vi "SetGlobalToZero.vi"(11 "subwindow control":T2={"2^n : x"=10, "2^n : y"=10, "lower left box Position"={"X"=1752.0, "Y"=1167.0}, "Height"=0, "Width"=0} {"Width" min=32 max=4704; "Height" min=2 max=3424; "2^n : y" min=1 max=13; "2^n : x" min=1 max=13}) -> ()   [LabVIEW 2018]
uses:
  <vilib>/Utility/miscctls.llb/LVPointDoubleTypeDef.ctl
  References.vi
  General Libraries/Photon Filtering.lvlib
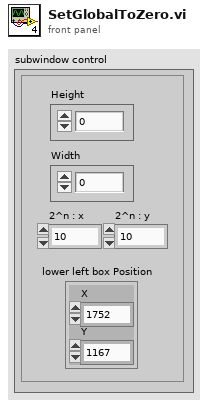
[diagram p1: front panel]
types:
  T1 = typedef "LVPointDoubleTypeDef.ctl" = cluster{"X":dbl, "Y":dbl}
  T2 = cluster{"2^n : x":i8, "2^n : y":i8, "lower left box Position":T1, "Height":i32, "Width":i32}
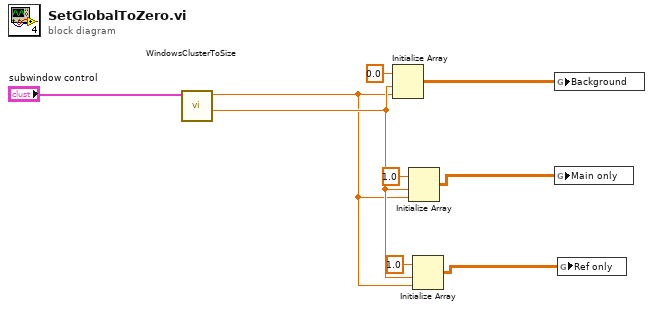
[diagram p0: block diagram]
diagram:
  n1 = call "WindowsClusterToSize.vi"("subwindow control 2"="subwindow control") -> ("Ny"=w6:dbl, "Nx"=w5:dbl)  [unwired: 9 in]
  n2 = Initialize Array(0.0 ("element"), w6, w5) -> (w7:dbl[][])
  n3 = Initialize Array "Initialize Array"(1.0 ("element"), w6, w5) -> (w2:dbl[][])
  n4 = Initialize Array "Initialize Array"(1.0 ("element"), w6, w5) -> (w1:dbl[][])
  n5 = global write "References.vi" "Background"(w7) -> ()
  n6 = global write "References.vi" "Main only"(w2) -> ()
  n7 = global write "References.vi" "Ref only"(w1) -> ()
